vi "Nov_24.vi"() -> ()   [LabVIEW 2020]
panel:
  out "?":dynamicdata(graph)
  out "?":dynamicdata(graph)
  out "?":dynamicdata(graph)
  in  "Motor Trottle":dbl(slide) scale=0.0..5.0
  out "Selected Signals":dynamicdata(graph)
  out "Signal Filtered":dynamicdata(graph)
  out "Motor":bool
  in  "Motor Enable":bool
  out "Swing":bool
  out "Hit 1":bool
  in  "Record Signal":bool
  in  "STOP":bool
  # "Gait Events"
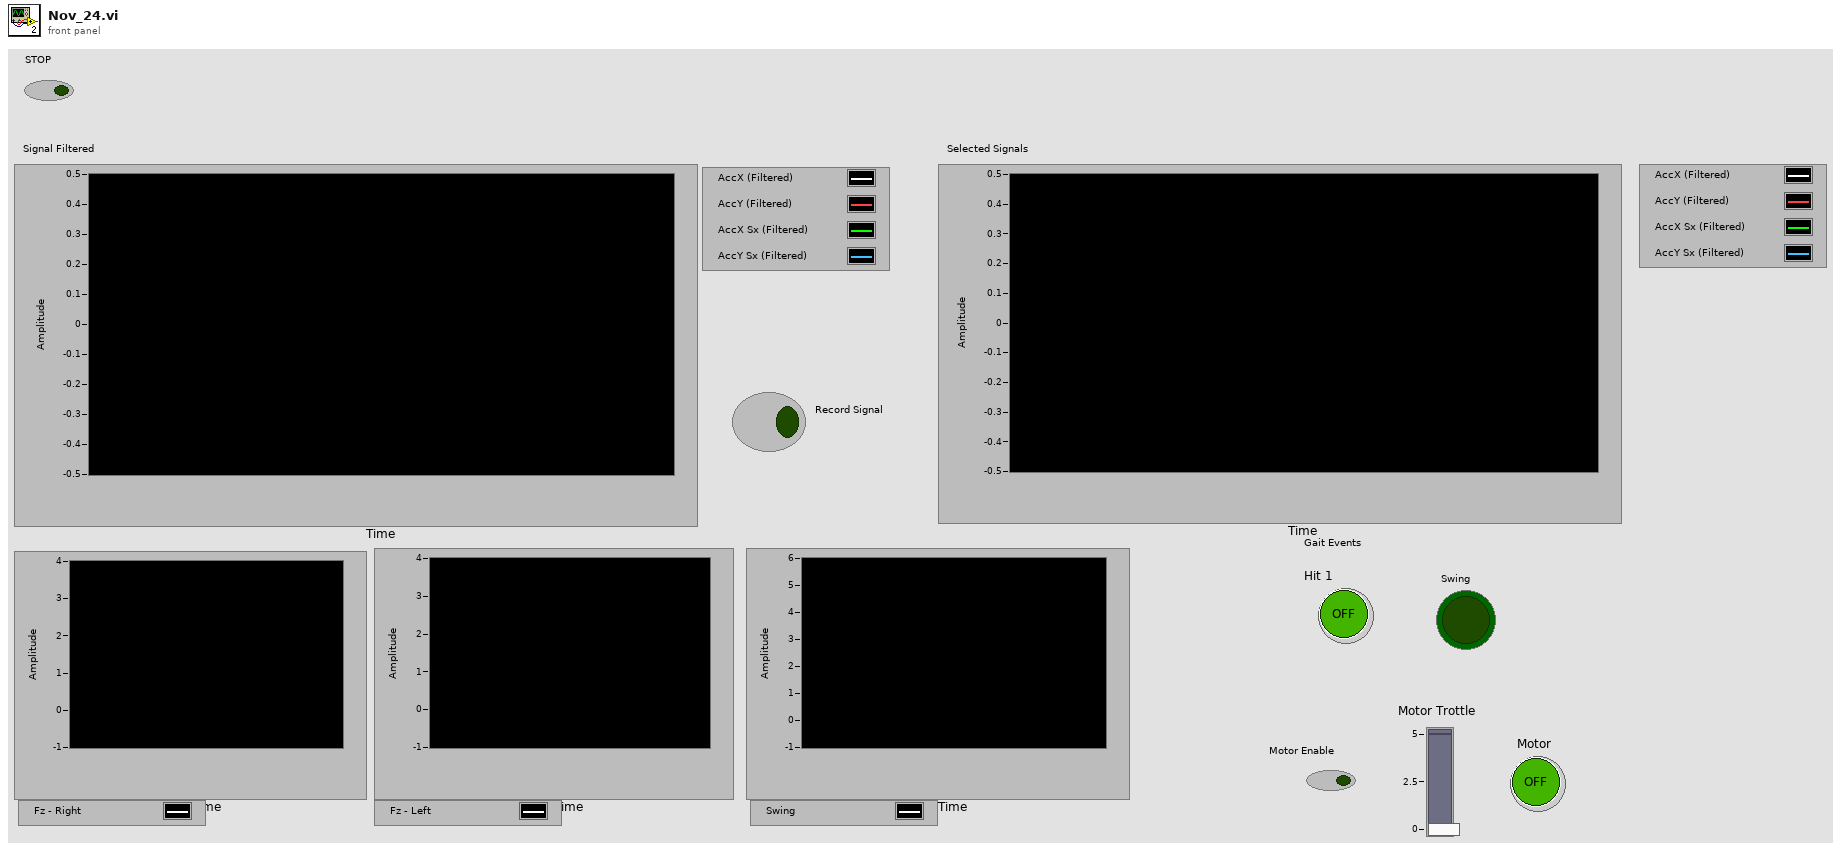
[diagram p1: front panel]
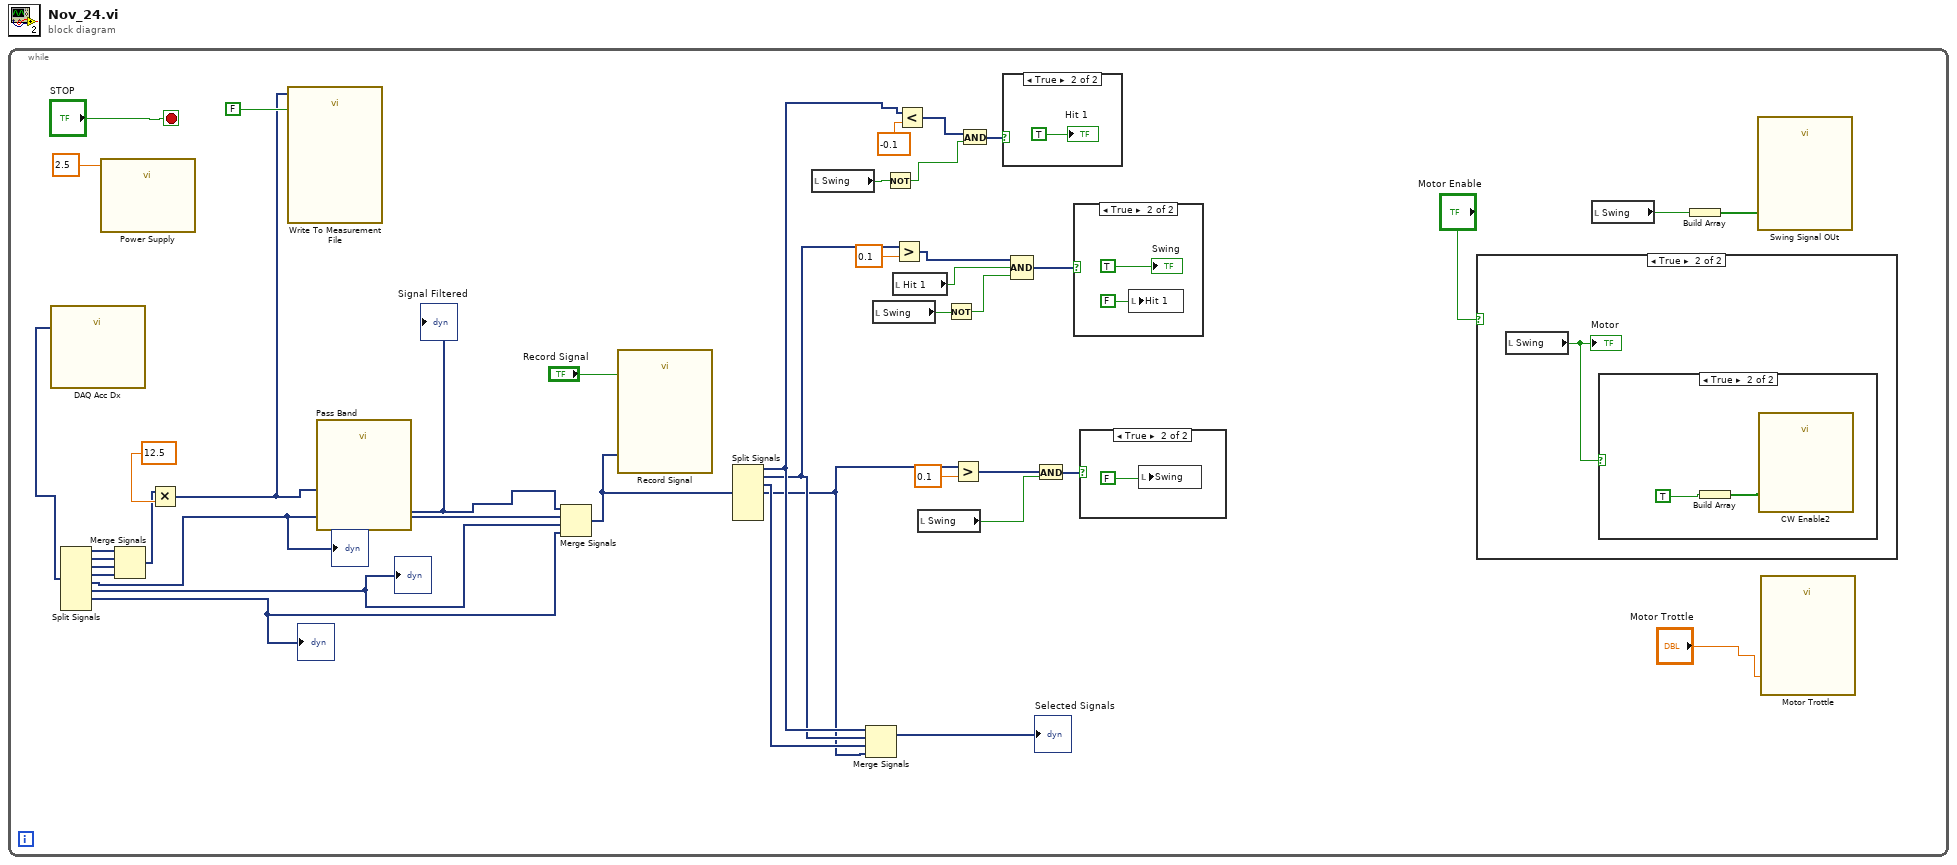
[diagram p0: block diagram]
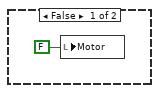
[diagram p3: hidden frame]
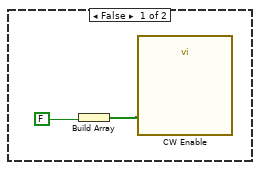
[diagram p4: hidden frame]
diagram:
  n1 = while {
    stop <- "STOP" stop-if-true
    n2 = call "DAQ Acc Dx"() -> ("data"=w28:dynamicdata)  [unwired: 16 in, 3 out]
    n3 = Split Signals(w28) -> (w27:dynamicdata, w26:dynamicdata, w5:dynamicdata, w4:dynamicdata, w3:dynamicdata, w2:dynamicdata, w1:dynamicdata)  [unwired: 8 in, 1 out]
    "?" <- w3
    "?" <- w2
    "?" <- w1
    n4 = call "Power Supply"("data"=2.5) -> ()  [unwired: 17 in, 2 out]
    n5 = Merge Signals(w27, w26, w5, w4) -> (w25:dynamicdata)
    n6 = Multiply(x=w25, y=12.5) -> (x*y=w29:dynamicdata)
    n7 = call "Write To Measurement File"("Signals"=w29, "Enable"=FALSE) -> ()  [unwired: 15 in, 3 out]
    n8 = call "Pass Band"("Signal"=w29) -> ("Filtered Signal"=w32:dynamicdata)  [unwired: 9 in, 1 out]
    "Signal Filtered" <- w32
    n9 = Merge Signals(w32, w3, w2, w1) -> (w31:dynamicdata)
    n10 = call "Record Signal"("Signals"=w31, "Enable"="Record Signal") -> ()  [unwired: 15 in, 3 out]
    n11 = Split Signals(w31) -> (w19:dynamicdata, w8:dynamicdata, w7:dynamicdata, w6:dynamicdata)  [unwired: 7 in, 3 out]
    n12 = local read "Swing"() -> (w24:bool)
    n13 = Merge Signals(w19, w8, w7, w6) -> (→"Selected Signals":dynamicdata)
    n14 = local read "Swing"() -> (w15:bool)
    n15 = Not(x=w24) -> (.not. x?=w23:bool)
    n16 = local read "Hit 1"() -> (w17:bool)
    n17 = Greater?(x=w8, y=0.1) -> (0:w16:dynamicdata)
    n18 = Less?(x=w19, y=-0.1) -> (x < y?=w18:dynamicdata)
    n19 = local read "Swing"() -> (w10:bool)
    n20 = Not(x=w15) -> (.not. x?=w14:bool)
    n21 = Greater?(x=w6, y=0.1) -> (0:w9:dynamicdata)
    n22 = And(x=w18, y=w23) -> (x .and. y?=w22:dynamicdata)
    n23 = case shown="True" w22 {
      frame False {
      }
      frame True {
        "Hit 1" <- TRUE
      }
    }
    n24 = Compound Arithmetic op=AND(w16, w17, w14) -> (w13:dynamicdata)
    n25 = And(x=w9, y=w10) -> (x .and. y?=w11:dynamicdata)
    n26 = case shown="True" w13 {
      frame False {
      }
      frame True {
        n27 = local write "Hit 1"(FALSE) -> ()
        "Swing" <- TRUE
      }
    }
    n28 = case shown="True" w11 {
      frame False {
      }
      frame True {
        n29 = local write "Swing"(FALSE) -> ()
      }
    }
    n30 = case shown="True" "Motor Enable" {
      frame False {
        n31 = local write "Motor"(FALSE) -> ()
      }
      frame True {
        n32 = local read "Swing"() -> (w45:bool)
        "Motor" <- w45
        n33 = case shown="True" w45 {
          frame False {
            n34 = Build Array(FALSE) -> (w47:bool[])
            n35 = call "CW Enable"("data"=w47) -> ()  [unwired: 17 in, 2 out]
          }
          frame True {
            n36 = Build Array "Build Array"(TRUE) -> (w48:bool[])
            n37 = call "CW Enable2"("data"=w48) -> ()  [unwired: 17 in, 2 out]
          }
        }
      }
    }
    n38 = local read "Swing"() -> (w34:bool)
    n39 = Build Array "Build Array"(w34) -> (w33:bool[])
    n40 = call "Swing Signal OUt"("data"=w33) -> ()  [unwired: 17 in, 2 out]
    n41 = call "Motor Trottle"("data"="Motor Trottle") -> ()  [unwired: 17 in, 2 out]
  }
